vi "FRIC_SerialPortGetPortName.vi"(8 "error in":errorcluster, 11 "Serial Port":T1) -> (0 "error out":errorcluster, 3 "VISA Refnum out":refnum<visa-resource-name>)   [LabVIEW 2016]
uses:
  <vilib>/Rock Robotics/WPI/SerialPort/WPI_SerialPort.ctl
panel:
  out "Hub Path":string[](array[string])
  out "OS Resource":string[](array[string])
  out "VISA Resource":string[](array[string])
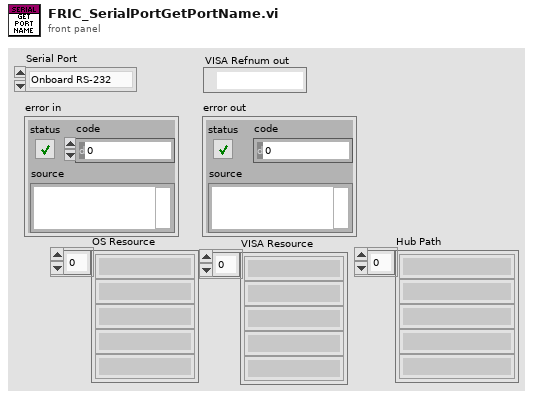
[diagram p1: front panel]
types:
  T1 = typedef "WPI_SerialPort.ctl" = enum16{"Onboard RS-232", "MXP TTL", "USB 1", "USB 2"}
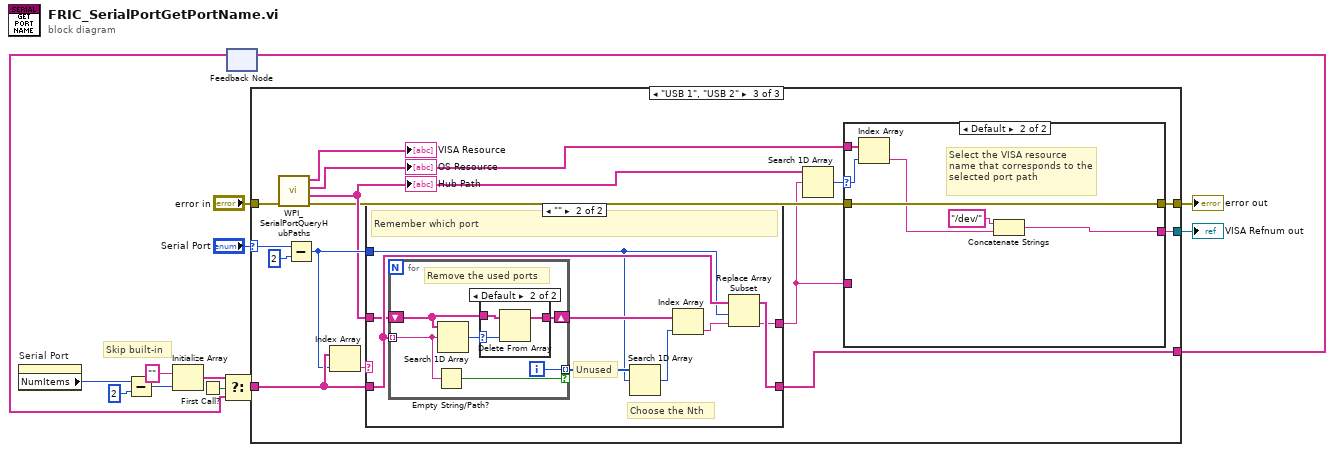
[diagram p0: block diagram]
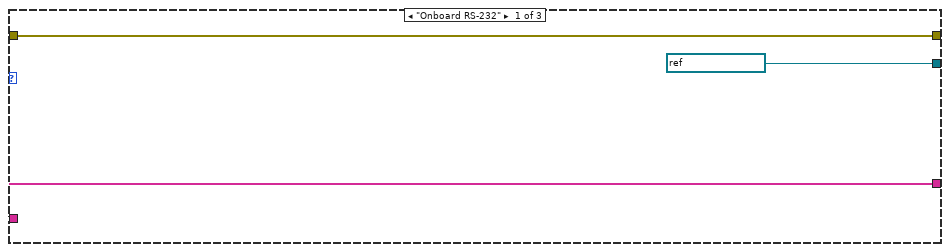
[diagram p2: hidden frame]
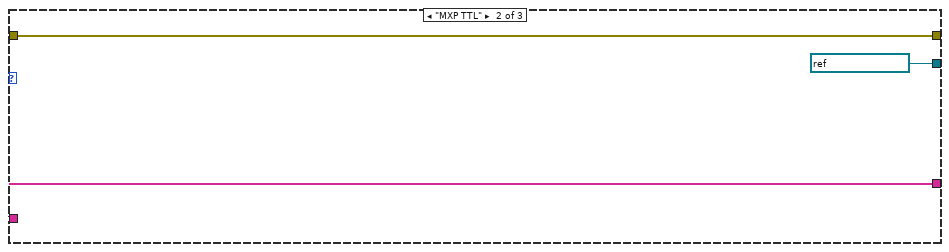
[diagram p3: hidden frame]
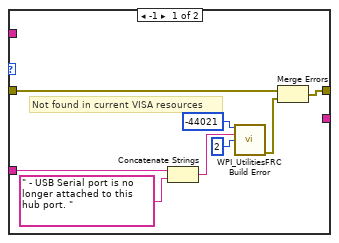
[diagram p4: hidden frame]
diagram:
  # "Skip built-in"
  n1 = property on="Serial Port" class="Enum (strict)"() -> ("NumItems"=w9:u32)  [unwired: 2 in, 2 out]
  n2 = Subtract(x=w9, y=u32 2 ("x")) -> (x-y=w2:u32)
  n3 = Initialize Array("", w2) -> (w7:string[])
  n4 = First Call?() -> (First Call?: T/F=w6:bool)
  n5 = feedback #1() -> (w5:string[])  [unwired: 1 in]
  n6 = Select(t=w7, s=w6, f=w5) -> (s? t:f=w4:string[])
  n7 = case shown="\"USB 1\", \"USB 2\"" "Serial Port" {
    selector: "Serial Port" -> [_ _ w30]
    tunnel: [refnum<visa-resource-name> "ASRL1::INSTR" ("VISA resource name") refnum<visa-resource-name> "ASRL2::INSTR" ("VISA resource name") w25] -> w13
    tunnel: "error in" -> [w15 w18 w34]
    tunnel: [w15 w18 w23] -> w10
    tunnel: w4 -> [w14 w17 w32]
    tunnel: [w14 w17 w28] -> w3
    frame "Onboard RS-232" {
    }
    frame "MXP TTL" {
    }
    frame "USB 1", "USB 2" {
      n8 = call <vilib>:"WPI_SerialPortQueryHubPaths.vi"("error in (no error)"=w34) -> ("error out"=w24:errorcluster, "Hub Path"=w27:string[], "OS Resource"=w20:string[], "VISA Resource"=→"VISA Resource":string[])  [unwired: 7 in]
      "OS Resource" <- w20
      "Hub Path" <- w27
      n9 = Subtract(x=w30, y=2 ("x")) -> (x-y=w29:i32)
      n10 = Index Array(array=w32, index=w29) -> (element=w33:string)
      n11 = case shown="\"\"" w33 {
        selector: w33 -> [w49 _]
        tunnel: w32 -> [w50 w55]
        tunnel: w27 -> [_ w52]
        tunnel: w29 -> [_ w54]
        tunnel: [w50 w53] -> w28
        tunnel: [w49 w51] -> w22
        frame Default {
          # "Previously assigned - just use it."
        }
        frame "" {
          # "Choose the Nth"
          # "Unused"
          # "Remember which port"
          n12 = for {
            tunnel: w55 -> [w62] mode=indexing
            tunnel: [w64] -> w58 mode=indexing if=w63
            shift-right: [w59] -> w57
            shift-left: w52 -> [w61]
            i -> [w64]
            # "Remove the used ports"
            n13 = Empty String/Path?(string/path=w62) -> (empty?=w63:bool)
            n14 = Search 1D Array(1D array=w61, element=w62) -> (index of element=w60:i32)  [unwired: 1 in]
            n15 = case shown="Default" w60 {
              selector: w60 -> [_ w67]
              tunnel: w61 -> [w65 w68]
              tunnel: [w65 w66] -> w59
              frame -1 {
              }
              frame Default {
                n16 = Delete From Array(array=w68, index=w67) -> (array with subset deleted=w66:string[])  [unwired: 1 in, 1 out]
              }
            }
          }
          n17 = Search 1D Array(1D array=w58, element=w54) -> (index of element=w56:i32)  [unwired: 1 in]
          n18 = Index Array(array=w57, index=w56) -> (element=w51:string)
          n19 = Replace Array Subset(array=w55, new element=w51, index=w54) -> (w53:string[])
        }
      }
      n20 = Search 1D Array(1D array=w27, element=w22) -> (index of element=w26:i32)  [unwired: 1 in]
      n21 = case shown="Default" w26 {
        selector: w26 -> [_ w48]
        tunnel: w20 -> [_ w47]
        tunnel: [_ w44] -> w25
        tunnel: [w41 w46] -> w23
        tunnel: w24 -> [w42 w46]
        tunnel: w22 -> [w36 _]
        frame -1 {
          # "Not found in current VISA resources"
          n22 = Concatenate Strings(w36, " - USB Serial port is no longer attached to this hub port. " ("extra error text")) -> (w37:string)
          n23 = call <vilib>:"WPI_UtilitiesFRC Build Error.vi"("error code"=-44021, "extra error text"=w37, "chain levels to remove (1)"=2) -> ("error out"=w35:errorcluster)  [unwired: 2 in, 10 out]
          n24 = Merge Errors(w42, w35) -> (w41:errorcluster)
        }
        frame Default {
          # "Select the VISA resource name that corresponds to the selected port path"
          n25 = Index Array(array=w47, index=w48) -> (element=w45:string)
          n26 = Concatenate Strings("/dev/" ("string"), w45) -> (w44:string)
        }
      }
    }
  }
  "VISA Refnum out" <- w13
  "error out" <- w10
  n27 = feedback-in #1(w3) -> ()
